vi "Rectangular Target - 2012.vi"() -> ()   [LabVIEW 2013]
doc: "This VI demonstrates how to do target processing on a laptop computer. It uses the same MJPG VI as the dashboard, sets a few of the important camera properties that impact processing, and carries out the same processing steps as the RT example also included in this project."
uses:
  <vilib>/Rock Robotics/WPI/Camera/WPI_CameraImageSize.ctl
  <vilib>/Rock Robotics/WPI/Camera/WPI_CameraWhite Balance Values.ctl
  <vilib>/vision/NI_Vision_Development_Module.lvlib
panel:
  in  "Camera Settings":T2={"FPS"=30, "Compression"=30, "Image Size"=enum."320x240"}
  in  "Camera IP Address":string="192.168.0.90"
  in  "Camera Type":enum16{"206", "1011"}(ring)
  out "Target Info":T3(array[cluster])
  in  "Area Size Limit":i32=444
  in  "Particle Count Limit":i32=10
  in  "Score Limits":T4={"Rect Coverage"=76.0, "Aspect Ratio"=70.0, "X Edge Strength"=40.0, "Y Edge Strength"=60.0}
  in  "Processing":enum32{"Color", "Intensity", "Intensity Open"}(tab)
  in  "Luminance":i32=255
  in  "Saturation":i32=255
  in  "Hue":i32(knob)=65 scale=0.0..255.0
  in  "Margins":cluster{"Hue":i32, "Sat":i32, "Lum":i32}={"Hue"=9, "Sat"=40, "Lum"=19} {"Sat" scale=0.0..40.0; "Lum" scale=0.0..40.0; "Hue" scale=0.0..40.0}
  in  "Range":cluster{"Lower value":sgl, "Upper value":sgl}={"Lower value"=150.0, "Upper value"=255.0} {"Lower value" scale=0.0..255.0; "Upper value" scale=0.0..255.0}
  in  "Range":cluster{"Lower value":sgl, "Upper value":sgl}={"Lower value"=150.0, "Upper value"=255.0} {"Lower value" scale=0.0..255.0; "Upper value" scale=0.0..255.0}
  in  "Annotate":bool=TRUE
  out "Processed Image":T5(plugin-control)
  out "Original Image":T5(plugin-control)
  # "Information:\nProcessing can be based on color or light intensity.\nParticles within the image are scored by rectangle coverage, aspect ratio, and\nfor being hollow with a bold edge. A particle is considered a target if all scores\nare above the score limits you set. Particles can be annotated -- surrounded by\na rectangle and scores drawn to the left .\nTo control the number of particles being scored, use the count limit and the size\nlimit.\nBe sure to set the Camera IP before running. The distance uses the camera type\nto index lens view angle."
  # "Click in the image to select target the color for processing."
  # "Green scores are above the limit, orange are below. Inner/outer rect\nindicates all passed."
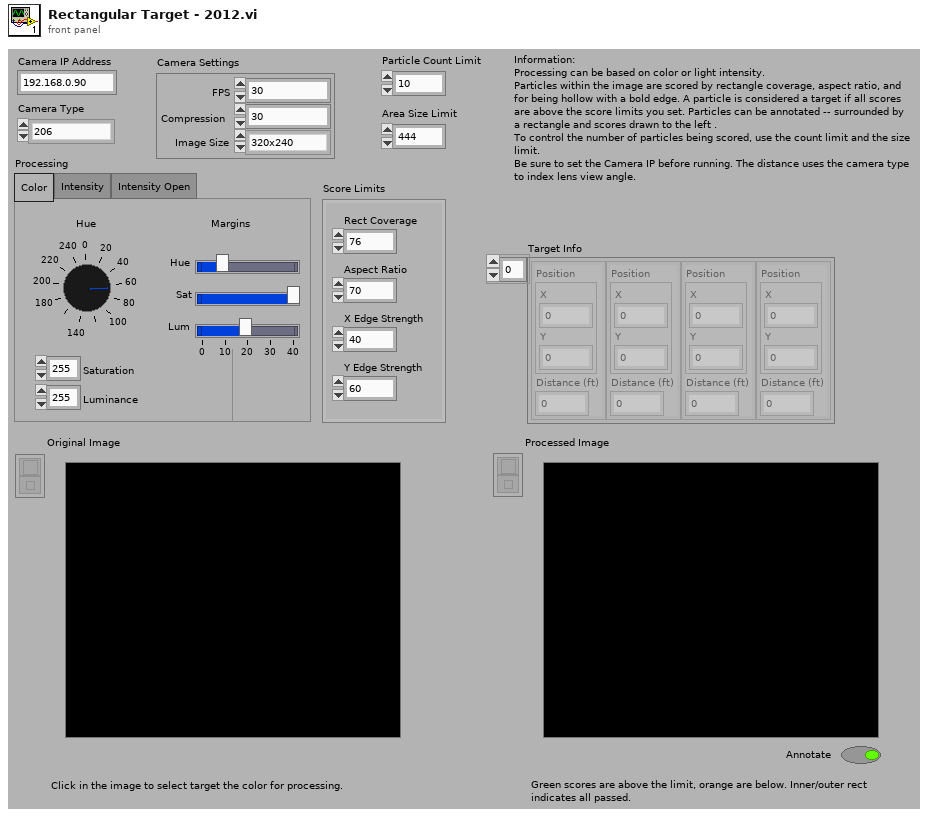
[diagram p1: front panel]
types:
  T1 = typedef "WPI_CameraImageSize.ctl" = enum16{"640x480", "320x240", "160x120"}
  T2 = cluster{"FPS":i32, "Compression":i32, "Image Size":T1}
  T3 = cluster{"Position":cluster{"X":dbl, "Y":dbl}, "Distance (ft)":dbl}[]
  T4 = cluster{"Rect Coverage":dbl, "Aspect Ratio":dbl, "X Edge Strength":dbl, "Y Edge Strength":dbl}
  T5 = typedef "IMAQ Image.ctl" = refnum<image>
  T6 = typedef "WPI_CameraWhite Balance Values.ctl" = enum16{"Auto", "Fixed indoor", "Fixed outdoor 1", "Fixed outdoor 2", "Fixed fluorescent 1", "Fixed fluorescent 2", "Hold current"}
  T7 = typedef "Image Type" = u32
  T8 = typedef "WPI_CameraDevRef.ctl" = cluster{"Camera Address":string, "CameraStatus":errorcluster, "Acquire Image Notifier":refnum<notifier>}
  T9 = enum32{"AutoM", "Close", "Dilate", "Erode", "Gradient", "Gradient out", "Gradient in", "Hit miss", "Open", "PClose", "POpen", "Thick", "Thin"}
  T10 = cluster{cluster{"Left":dbl, "Top":dbl, "Right":dbl, "Bottom":dbl}, dbl[]}[]
  T11 = cluster{"Left":dbl, "Top":dbl, "Right":dbl, "Bottom":dbl}
  T12 = cluster{"Target Center (-1 to 1)":cluster{"X":dbl, "Y":dbl}, "Distance (ft)":dbl}
  T13 = cluster{"Target Center (-1 to 1)":cluster{"X":dbl, "Y":dbl}, "Distance (ft)":dbl}[]
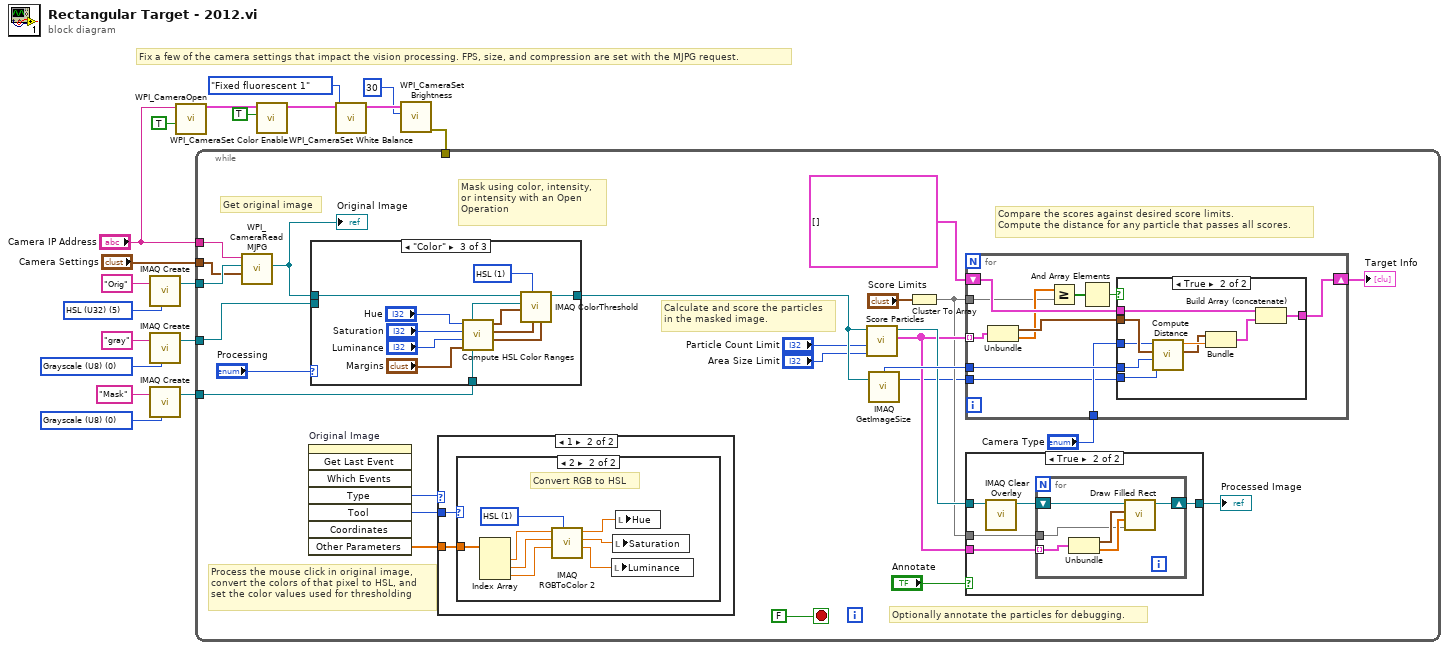
[diagram p0: block diagram]
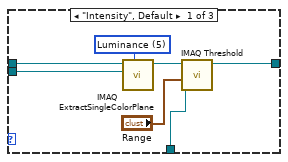
[diagram p3: hidden frame]
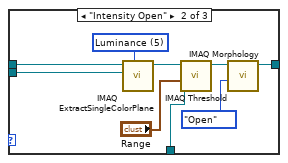
[diagram p4: hidden frame]
diagram:
  w12 = T7 0 items=["Grayscale (U8)", "Grayscale (I16)", "Grayscale (SGL)", "Complex (CSG)", "RGB (U32)", "HSL (U32)", "RGB (U64)", "Grayscale (U16)"] ("Image Type")
  w16 = T7 5 items=["Grayscale (U8)", "Grayscale (I16)", "Grayscale (SGL)", "Complex (CSG)", "RGB (U32)", "HSL (U32)", "RGB (U64)", "Grayscale (U16)"] ("Image Type")
  w19 = T7 0 items=["Grayscale (U8)", "Grayscale (I16)", "Grayscale (SGL)", "Complex (CSG)", "RGB (U32)", "HSL (U32)", "RGB (U64)", "Grayscale (U16)"] ("Image Type")
  # "Fix a few of the camera settings that impact the vision processing. FPS, size, and compression are set with the MJPG request."
  n1 = call "IMAQ Create"("Image Name"="Orig", "Image Type"=w16) -> ("New Image"=w15:T5)  [unwired: 2 in, 2 out]
  n2 = call "IMAQ Create"("Image Name"="gray", "Image Type"=w19) -> ("New Image"=w14:T5)  [unwired: 2 in, 2 out]
  n3 = call "IMAQ Create"("Image Name"="Mask", "Image Type"=w12) -> ("New Image"=w11:T5)  [unwired: 2 in, 2 out]
  n4 = call <vilib>:"WPI_CameraOpen.vi"("Disallow Simulation"=TRUE, "Camera Address"="Camera IP Address") -> ("CameraDevRef"=w9:T8)  [unwired: 8 in, 1 out]
  n5 = call <vilib>:"WPI_CameraSet Color Enable.vi"("Color Enabled"=TRUE, "CameraDevRef"=w9) -> ("CameraDevRef Out"=w7:T8)  [unwired: 8 in, 1 out]
  n6 = call <vilib>:"WPI_CameraSet White Balance.vi"("White Balance"=WPI_CameraWhite_Balance_Values."Fixed fluorescent 1", "CameraDevRef"=w7) -> ("CameraDevRef Out"=w5:T8)  [unwired: 8 in, 1 out]
  n7 = call <vilib>:"WPI_CameraSet Brightness.vi"("Brightness"=30, "CameraDevRef"=w5) -> ("error out"=w3:errorcluster)  [unwired: 8 in, 1 out]
  n8 = while {
    tunnel: w15 -> [w35]
    tunnel: w14 -> [w44]
    tunnel: w11 -> [w43]
    tunnel: "Camera IP Address" -> [w33]
    tunnel: w3 -> [_]
    tunnel: "Camera Settings" -> [w20]
    stop <- FALSE stop-if-true
    # "Optionally annotate the particles for debugging."
    # "Compare the scores against desired score limits.\nCompute the distance for any particle that passes all scores."
    # "Process the mouse click in original image,\nconvert the colors of that pixel to HSL, and\nset the color values used for thresholding"
    # "Calculate and score the particles\nin the masked image."
    # "Mask using color, intensity,\nor intensity with an Open\nOperation"
    # "Get original image"
    n9 = call <vilib>:"WPI_CameraRead MJPG.vi"("Camera Settings"=w20, "Image"=w35, "address"=w33) -> ("Image Out"=w34:T5)  [unwired: 6 in, 2 out]
    "Original Image" <- w34
    n10 = invoke on="Original Image" class="ImageControl" method="Get Last Event"() -> ("Type"=w37:i32, "Tool"=w38:i32, "Other Parameters"=w39:sgl[])  [unwired: 8 in, 5 out]
    n11 = case shown="\"Color\"" "Processing" {
      tunnel: w34 -> [w63 w72 w83]
      tunnel: w44 -> [w62 w71 _]
      tunnel: w43 -> [w60 w69 w82]
      tunnel: [w58 w65 w81] -> w25
      frame "Intensity", Default {
        w57 = 5 items=["Red", "Green", "Blue", "Hue", "Saturation", "Luminance", "Value", "Intensity"] ("Color Plane")
        n12 = call "IMAQ ExtractSingleColorPlane"("Color Plane"=w57, "Image Dst"=w62, "Image Src"=w63) -> ("Image Dst Out"=w61:T5)  [unwired: 1 in, 7 out]
        n13 = call "IMAQ Threshold"("Range"="Range", "Image Dst"=w60, "Image Src"=w61) -> ("Image Dst Out"=w58:T5)  [unwired: 3 in, 5 out]
      }
      frame "Intensity Open" {
        w64 = 5 items=["Red", "Green", "Blue", "Hue", "Saturation", "Luminance", "Value", "Intensity"] ("Color Plane")
        n14 = call "IMAQ ExtractSingleColorPlane"("Color Plane"=w64, "Image Dst"=w71, "Image Src"=w72) -> ("Image Dst Out"=w70:T5)  [unwired: 1 in, 7 out]
        n15 = call "IMAQ Threshold"("Range"="Range", "Image Dst"=w69, "Image Src"=w70) -> ("Image Dst Out"=w66:T5)  [unwired: 3 in, 5 out]
        n16 = call "IMAQ Morphology"("Operation"=T9."Open", "Image Src"=w66) -> ("Image Dst Out"=w65:T5)  [unwired: 8 in, 1 out]
      }
      frame "Color" {
        w80 = u16 1 items=["RGB", "HSL", "HSV", "HSI"] ("Color Mode")
        n17 = call "Compute HSL Color Ranges.vi"("Margins"="Margins", "Luminance"="Luminance", "Saturation"="Saturation", "Hue"="Hue") -> ("Lum Range"=w77:cluster{i32, i32}, "Sat Range"=w78:cluster{i32, i32}, "Hue Range"=w79:cluster{i32, i32})  [unwired: 5 in]
        n18 = call "IMAQ ColorThreshold"("Blue or Luma or Val or Inten Range"=w77, "Green or Sat Range"=w78, "Color Mode"=w80, "Red or Hue Range"=w79, "Image Dst"=w82, "Image Src"=w83) -> ("Image Dst Out"=w81:T5)  [unwired: 4 in, 1 out]
      }
    }
    n19 = case shown="1" w37 {
      tunnel: w38 -> [_ w106]
      tunnel: w39 -> [_ w105]
      frame 0, Default {
      }
      frame 1 {
        n20 = case shown="2" w106 {
          tunnel: w105 -> [_ w114]
          frame Default {
          }
          frame 2 {
            w113 = u16 1 items=["RGB", "HSL", "HSV", "HSI", "CIE L*a*b*", "CIE XYZ"] ("Color Mode")
            # "Convert RGB to HSL"
            n21 = Index Array(array=w114) -> (element #1=w112:sgl, element #2=w110:sgl, element #3=w108:sgl)  [unwired: 3 in]
            n22 = call "IMAQ RGBToColor 2"("Color Mode"=w113, "Blue value"=w108, "Green value"=w110, "Red value"=w112) -> ("Blue or Luma or Val or Inten or Z or b*value"=w107:dbl, "Green or Sat or Y or a* value"=w109:dbl, "Red or Hue or X or L* value"=w111:dbl)  [unwired: 4 in, 1 out]
            n23 = local write "Luminance"(w107) -> ()
            n24 = local write "Saturation"(w109) -> ()
            n25 = local write "Hue"(w111) -> ()
          }
        }
      }
    }
    n26 = call "Score Particles.vi"("Area Size Limit"="Area Size Limit", "Particle Count Limit"="Particle Count Limit", "Image Refnum in"=w25) -> ("Scored Particle Info"=w28:T10, "Image Refnum out"=w32:T5)  [unwired: 7 in]
    n27 = call "IMAQ GetImageSize"("Image"=w25) -> ("Y Resolution"=w21:i32, "X Resolution"=w36:i32)  [unwired: 3 in, 1 out]
    n28 = Cluster To Array(cluster="Score Limits") -> (array=w26:dbl[])
    n29 = for {
      shift-right: [w93] -> w40
      shift-left: T3 [] -> [w94]
      tunnel: w36 -> [w92]
      tunnel: w28 -> [w90] mode=indexing
      tunnel: w26 -> [w85]
      tunnel: "Camera Type" -> [w89]
      tunnel: w21 -> [w84]
      n30 = Unbundle(w90) -> (w91:T11, w86:dbl[])
      n31 = Greater Or Equal?(x=w86, y=w85) -> (x >= y?=w88:bool[])
      n32 = And Array Elements(Boolean array=w88) -> (logical AND=w87:bool)
      n33 = case shown="True" w87 {
        tunnel: w94 -> [w95 w104]
        tunnel: [w95 w103] -> w93
        tunnel: w91 -> [_ w99]
        tunnel: w92 -> [_ w101]
        tunnel: w89 -> [_ w98]
        tunnel: w84 -> [_ w96]
        frame False {
        }
        frame True {
          n34 = call "Compute Distance.vi"("Y Image Resolution"=w96, "X Image Resolution"=w101, "Bounding Box"=w99, "Camera Type"=w98) -> ("Target Center (-1 to 1)"=w97:cluster{"X":dbl, "Y":dbl}, "Distance (ft)"=w100:dbl)  [unwired: 6 in]
          n35 = Bundle("Target Center (-1 to 1)"=w97, "Distance (ft)"=w100) -> (w102:T12)  [unwired: 1 in]
          n36 = Build Array (concatenate)(w104, w102) -> (w103:T13)
        }
      }
    }
    "Target Info" <- w40
    n37 = case shown="True" "Annotate" {
      tunnel: w32 -> [w45 w50]
      tunnel: [w45 w49] -> w29
      tunnel: w28 -> [_ w47]
      tunnel: w26 -> [_ w46]
      frame False {
      }
      frame True {
        n38 = call "IMAQ Clear Overlay"("Image"=w50) -> ("Image Out"=w48:T5)  [unwired: 2 in, 8 out]
        n39 = for {
          shift-right: [w55] -> w49
          shift-left: w48 -> [w56]
          tunnel: w47 -> [w52] mode=indexing
          tunnel: w46 -> [w51]
          n40 = Unbundle(w52) -> (w53:T11, w54:dbl[])
          n41 = call "Draw Filled Rect.vi"("Limits"=w51, "Scores"=w54, "Bounding Box"=w53, "image in"=w56) -> ("image out"=w55:T5)  [unwired: 7 in]
        }
      }
    }
    "Processed Image" <- w29
  }
